vi "Run.vi"(8 "error in (no error)":errorcluster caption="entrée d'erreur (pas d'erreur)", 10 "y":string[][](array[string]), 11 "label_binarize.lvclass":refnum<class "label_binarize.lvclass">) -> (0 "error out":errorcluster caption="sortie d'erreur", 2 "Data":T1, 3 "label_binarize.lvclass":refnum<class "label_binarize.lvclass">)   [LabVIEW 2020, in "label_binarize.lvclass"]
doc: "Returns : \n\n- Y : numpy array or CSR matrix of shape [n_samples, n_classes]\nShape will be [n_samples, 1] for binary problems."
uses:
  label_binarize.lvclass
  label_binarize.lvclass/label_binarize.ctl
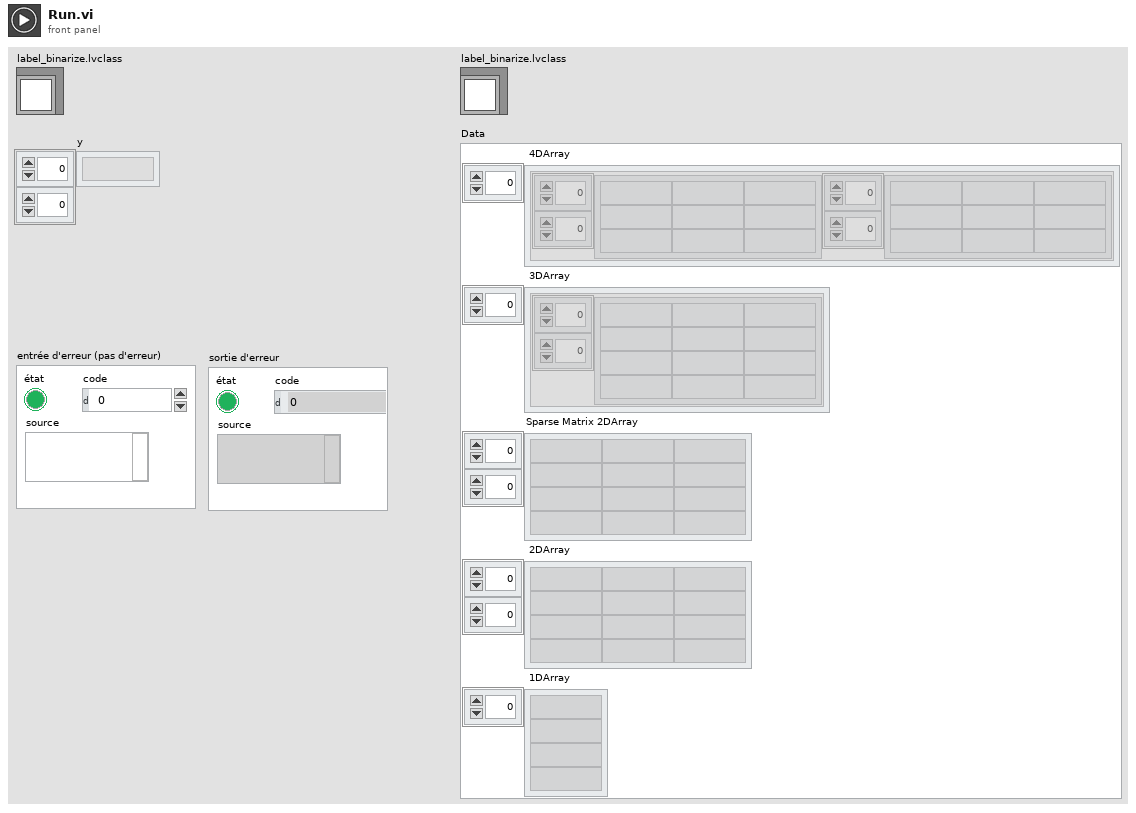
[diagram p1: front panel]
types:
  T1 = cluster{" 4DArray":cluster{"1":string[][], "2":string[][]}[], " 3DArray":cluster{"Tableau":string[][]}[], "Sparse Matrix 2DArray":string[][], " 2DArray":string[][], " 1DArray":string[]}
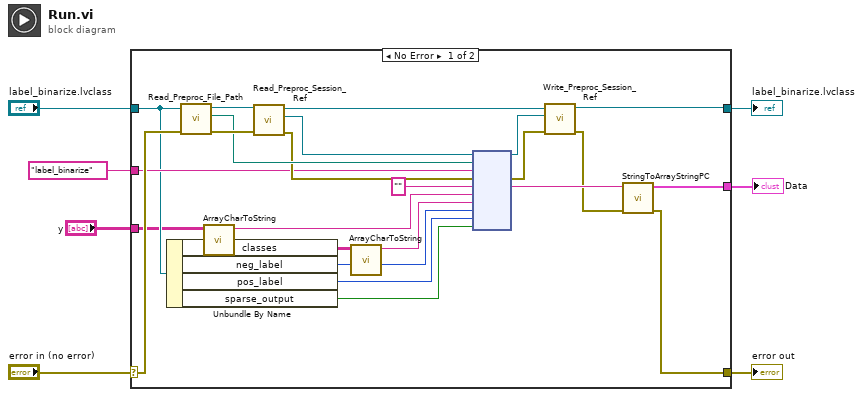
[diagram p0: block diagram]
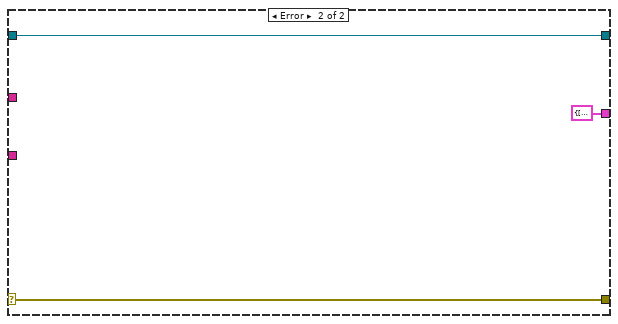
[diagram p2: hidden frame]
diagram:
  n1 = case shown="No Error" "error in (no error)" {
    selector: "error in (no error)" -> [w21 w34]
    tunnel: [w12 w34] -> w6
    tunnel: [w16 w33] -> w4
    tunnel: "label_binarize.lvclass" -> [w19 w33]
    tunnel: "label_binarize" ("Fonction") -> [w20 _]
    tunnel: [w13 T1 {" 4DArray"=[], " 3DArray"=[], "Sparse Matrix 2DArray"=[], " 2DArray"=[], " 1DArray"=[]} ("Data")] -> w1
    tunnel: "y" -> [w11 _]
    frame No Error {
      n2 = Unbundle By Name(w19) -> ("classes"=w9:string[][], "neg_label"=w22:i32, "pos_label"=w18:i32, "sparse_output"=w17:bool)
      n3 = call-dynamic "Read_Preproc_File_Path.vi"("error in (no error)"=w21, "Python in"=w19) -> ("error out"=w30:errorcluster, "File_Path"=w27:path, "Python out"=w31:refnum<class "label_binarize.lvclass">)  [unwired: 7 in]
      n4 = call "ArrayCharToString.vi"("TAB"=w11) -> ("Instruction"=w10:string)  [unwired: 10 in]
      n5 = call-dynamic "Read_Preproc_Session_Ref.vi"("error in (no error)"=w30, "Python in"=w31) -> ("error out"=w26:errorcluster, "Session_ref"=w28:refnum<k35>, "Python out"=w29:refnum<class "label_binarize.lvclass">)  [unwired: 7 in]
      n6 = call "ArrayCharToString.vi"("TAB"=w9) -> ("Instruction"=w8:string)  [unwired: 10 in]
      n7 = node(w28, w27, w20, w26, "", w10, w8, w22, w18, w17) -> (w24:refnum<k35>, w25:errorcluster, w15:string)  [unwired: 5 in, 2 out]
      n8 = call-dynamic "Write_Preproc_Session_Ref.vi"("error in (no error)"=w25, "Session_ref"=w24, "Python in"=w29) -> ("error out"=w14:errorcluster, "Python out"=w16:refnum<class "label_binarize.lvclass">)  [unwired: 7 in]
      n9 = call "StringToArrayStringPC.vi"("sortie d'erreur"=w14, "Return value"=w15) -> ("sortie d'erreur"=w12:errorcluster, "Data"=w13:T1)  [unwired: 8 in]
    }
    frame Error {
    }
  }
  "error out" <- w6
  "label_binarize.lvclass" <- w4
  "Data" <- w1
